vi "observer.vi"(2 "x 2":dbl, 3 "x_1":dbl, 4 "Measured Speed":dbl) -> (0 "Estimated acceleration":dbl, 1 "Estimated speed":dbl)   [LabVIEW 2023]
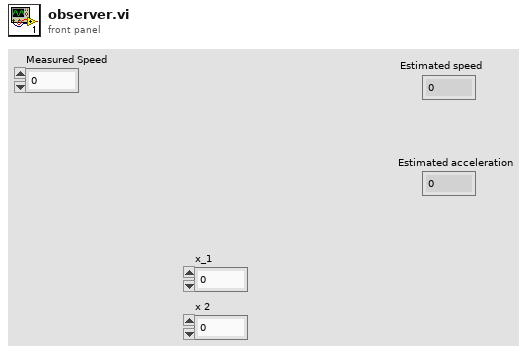
[diagram p1: front panel]
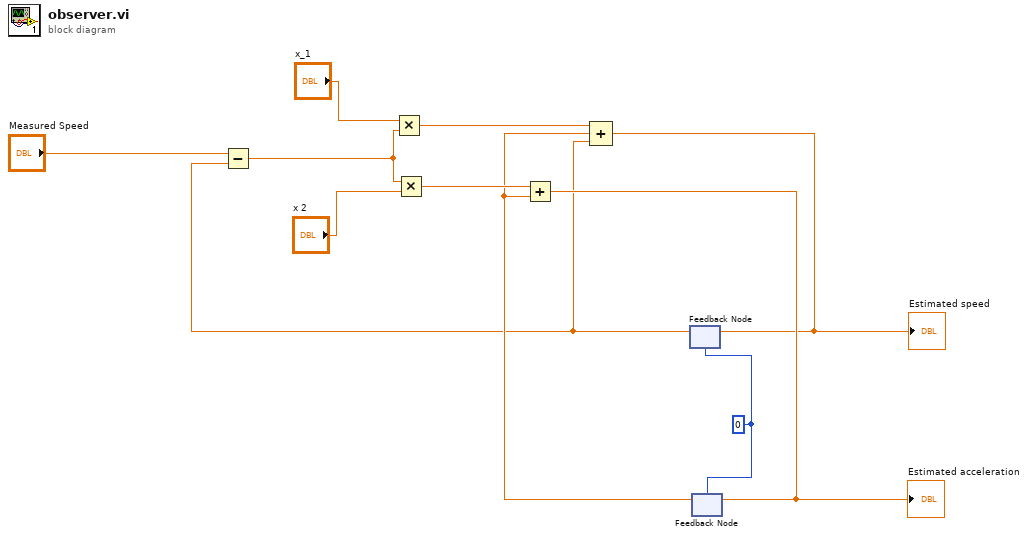
[diagram p0: block diagram]
diagram:
  w11 = 0
  n1 = feedback #1(w11) -> (w2:dbl)
  n2 = Subtract(x="Measured Speed", y=w2) -> (x-y=w7:dbl)
  n3 = Multiply(x="x_1", y=w7) -> (x*y=w4:dbl)
  n4 = Multiply(x=w7, y="x 2") -> (x*y=w6:dbl)
  n5 = feedback #2(w11) -> (w3:dbl)
  n6 = Add(x=w6, y=w3) -> (x+y=w5:dbl)
  "Estimated acceleration" <- w5
  n7 = Compound Arithmetic op=ADD(w4, w3, w2) -> (w1:dbl)
  "Estimated speed" <- w1
  n8 = feedback-in #1(w1) -> ()
  n9 = feedback-in #2(w5) -> ()
